vi "choose type of cal file to save.vi"(8 "error in (no error)":errorcluster) -> (0 "error out":errorcluster, 3 "double precision float":u8)   [LabVIEW 2014, in "AvaSpec.lvlib" / "AvaSpec Logging.lvlib"]
uses:
  AvaSpec Logging.lvlib
panel:
  in  "OK Button":bool
  in  "Radio Buttons":T1(radio)
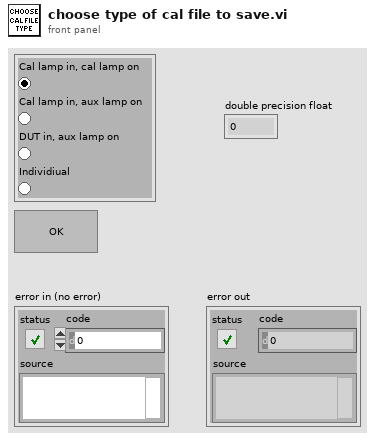
[diagram p1: front panel]
types:
  T1 = enum32{"Cal lamp in, cal lamp on", "Cal lamp in, aux lamp on", "DUT in, aux lamp on", "Individiual"}
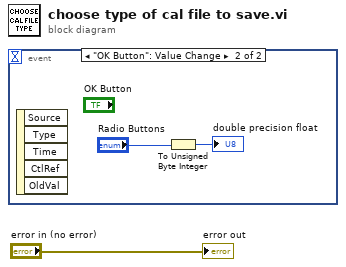
[diagram p0: block diagram]
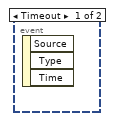
[diagram p2: hidden frame]
diagram:
  n1 = event shown="[1] \"OK Button\": Value Change" {
    selector: _ -> [_ _]
    dyn-events: _ -> [_ _]
    timeout: _ -> [_ _]
    event Timeout {
      n2 = event-data() -> ()  [unwired: 1 in, 3 out]
    }
    event "OK Button": Value Change {
      n3 = event-data() -> ()  [unwired: 1 in, 5 out]
      n4 = To Unsigned Byte Integer(number="Radio Buttons") -> (unsigned 8bit integer=→"double precision float":u8)
    }
  }
  "error out" <- "error in (no error)"
